vi "Create Group.vi"(8 "error in (no error)":errorcluster, 10 "Group":string, 11 "PrefsDB in":refnum<class "PrefsDB.lvclass">) -> (0 "error out":errorcluster, 2 "Pref Group":refnum<class "Pref Group.lvclass">, 3 "PrefsDB out":refnum<class "PrefsDB.lvclass">)   [LabVIEW 2023, in "User Prefs.lvlib" / "PrefsDB.lvclass"]
uses:
  PrefsDB.lvclass
  Pref Group/Pref Group.lvclass
  PrefsDB.lvclass/PrefsDB.ctl
  Pref Group.ctl
  lv-cdm/CDM-Config/Config Manager/Config Manager.lvclass
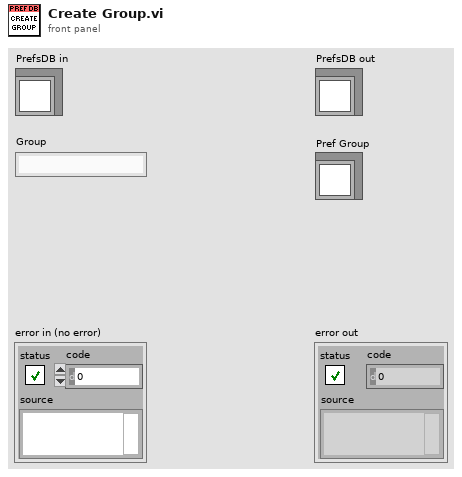
[diagram p1: front panel]
types:
  T1 = typedef "User Prefs.lvlib/PrefsDB.lvclass/Pref Group.ctl" = cluster{"Config Manager":refnum<class "Config Manager.lvclass">, "Group":string}
  T2 = typedef "User Prefs.lvlib/PrefsDB.lvclass/Ref Data.ctl" = cluster{"Map":map{string, T1}}
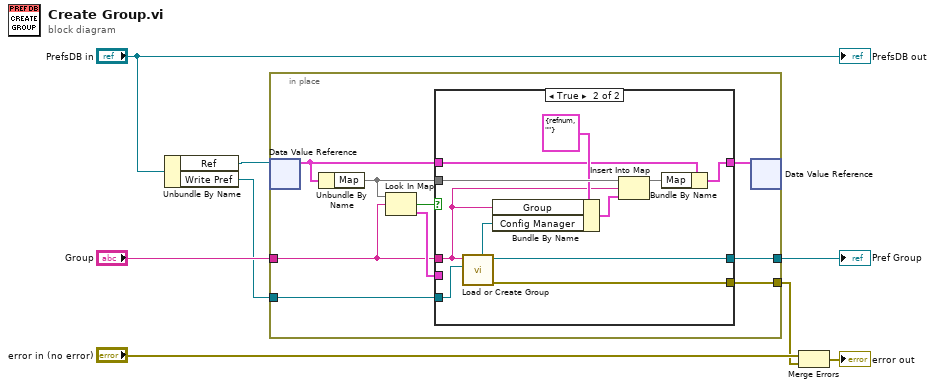
[diagram p0: block diagram]
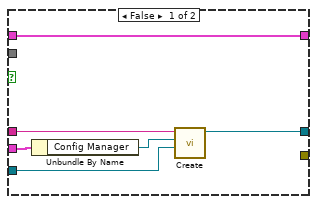
[diagram p2: hidden frame]
diagram:
  n1 = Unbundle By Name("PrefsDB in") -> ("Ref"=w6:refnum<data-value>, "Write Pref"=w1:refnum<user-event>)
  n2 = in-place {
    in-place-border: "Group" -> [w15]
    in-place-border: [w14] -> w4
    in-place-border: [w10] -> w2
    in-place-border: w1 -> [w9]
    n3 = in-place-dvr #1(w6) -> (w12:T2)  [unwired: 1 out]
    n4 = Unbundle By Name(w12) -> ("Map"=w11:map{string, T1})
    n5 = Look In Map(map=w11, key=w15) -> (key not found?=w17:bool, value=w16:T1)  [unwired: 1 in]
    n6 = case shown="True" w17 {
      tunnel: w16 -> [w23 _]
      tunnel: w15 -> [w22 w28]
      tunnel: [w20 w26] -> w14
      tunnel: [w19 w29] -> w13
      tunnel: w12 -> [w19 w31]
      tunnel: w11 -> [_ w34]
      tunnel: [_ w25] -> w10
      tunnel: w9 -> [w18 w24]
      frame False {
        n7 = Unbundle By Name(w23) -> ("Config Manager"=w21:refnum<class "Config Manager.lvclass">)
        n8 = call "Create.vi"("Write Pref"=w18, "Config Manager"=w21, "Group"=w22) -> ("Pref Group out"=w20:refnum<class "Pref Group.lvclass">)  [unwired: 7 in, 1 out]
      }
      frame True {
        n9 = call "Load or Create Group.vi"("Write Pref"=w24, "Group Name"=w28) -> ("error out"=w25:errorcluster, "Pref Group"=w26:refnum<class "Pref Group.lvclass">, "Config Manager"=w27:refnum<class "Config Manager.lvclass">)  [unwired: 7 in]
        n10 = Bundle By Name(cluster=T1 {"Config Manager"=refnum, "Group"=""} ("value"), "Group"=w28, "Config Manager"=w27) -> (w32:T1)
        n11 = Insert Into Map(map in=w34, key=w28, value=w32) -> (map out=w30:map{string, T1})  [unwired: 2 out]
        n12 = Bundle By Name(cluster=w31, "Map"=w30) -> (w29:T2)
      }
    }
    n13 = in-place-dvr #1(w13) -> ()  [unwired: 2 out]
  }
  "Pref Group" <- w4
  n14 = Merge Errors("error in (no error)", w2) -> (→"error out":errorcluster)
  "PrefsDB out" <- "PrefsDB in"
